vi "Measure.vi"(6 "Init work":bool, 7 "Update period":dbl, 8 "error in (no error)":errorcluster, 9 "Last request":bool, 10 "Requester":string, 11 "Format Resonances in":refnum<class "Format Resonances.lvclass">) -> (0 "error out":errorcluster, 3 "Format Resonances out":refnum<class "Format Resonances.lvclass">)   [LabVIEW 2024, in "Format Resonances.lvclass"]
uses:
  Format Resonances.lvclass
  Format Resonances.lvclass/Format Resonances.ctl
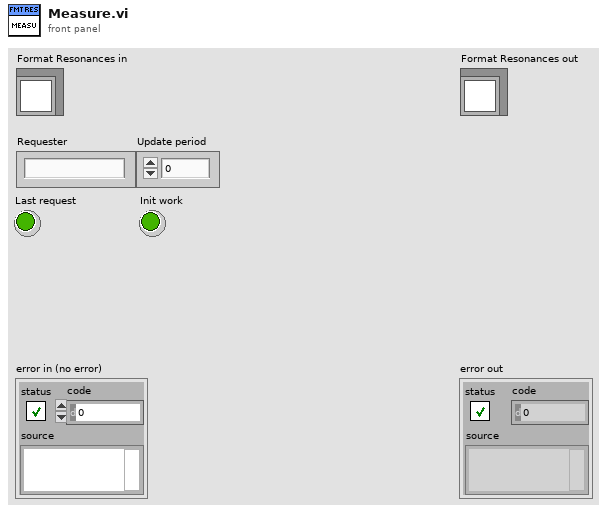
[diagram p1: front panel]
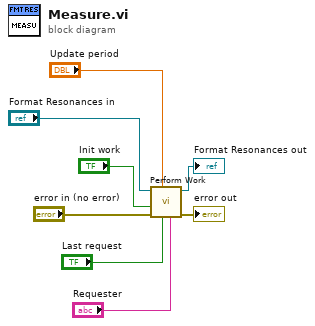
[diagram p0: block diagram]
diagram:
  n1 = call-dynamic "Perform Work.vi"("Controller name"="Requester", "Last request"="Last request", "Update period"="Update period", "error in (no error)"="error in (no error)", "Initialize"="Init work", "Measure Object in"="Format Resonances in") -> ("error out"=→"error out":errorcluster, "Measure Object out"=→"Format Resonances out":refnum<class "Format Resonances.lvclass">)  [unwired: 4 in]
